vi "writeNumberOfImagesXML.vi"(8 "error in (no error)":errorcluster, 10 "NativeXML in":refnum<class "NativeXML.lvclass">, 11 "WinX32Settings in":refnum<class "WinX32Settings.lvclass">) -> (0 "error out":errorcluster, 2 "NativeXML out":refnum<class "NativeXML.lvclass">, 3 "WinX32Settings out":refnum<class "WinX32Settings.lvclass">)   [LabVIEW 2011, in "Tools.lvlib" / "Settings.lvlib" / "WinX32Settings.lvclass"]
uses:
  WinX32Settings.lvclass
  NativeXML/NativeXML.lvclass
  WinX32Settings.lvclass/WinX32Settings.ctl
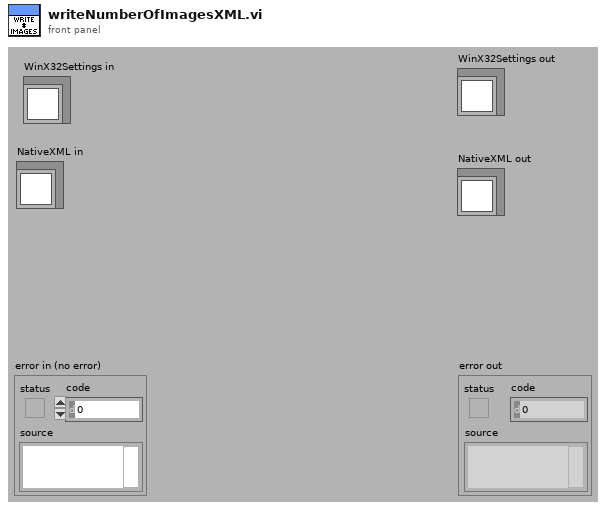
[diagram p1: front panel]
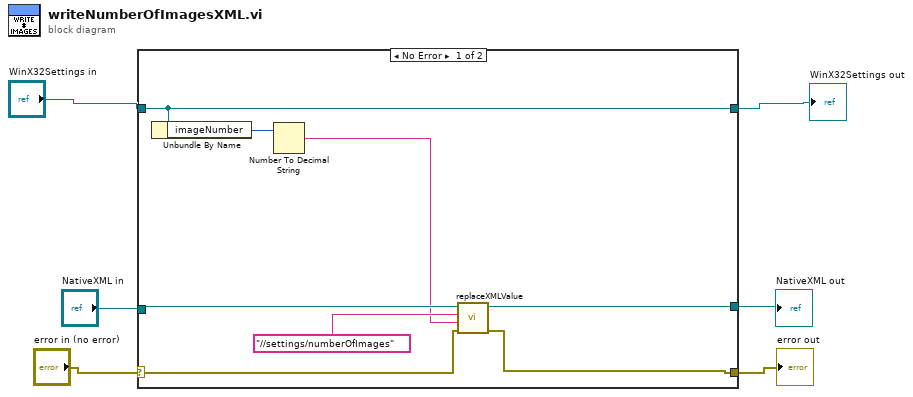
[diagram p0: block diagram]
diagram:
  n1 = case shown="No Error" "error in (no error)" {
    selector: "error in (no error)" -> [w10 w17]
    tunnel: [w9 w17] -> w6
    tunnel: [w14 w16] -> w1
    tunnel: "WinX32Settings in" -> [w14 w16]
    tunnel: "NativeXML in" -> [w13 w15]
    tunnel: [w12 w15] -> w5
    frame No Error {
      n2 = Unbundle By Name(w14) -> ("imageNumber"=w8:i32)
      n3 = Number To Decimal String(number=w8) -> (decimal integer string=w7:string)  [unwired: 1 in]
      n4 = call "replaceXMLValue.vi"("error in (no error)"=w10, "value"=w7, "replace in"="//settings/numberOfImages", "NativeXML in"=w13) -> ("error out"=w9:errorcluster, "NativeXML out"=w12:refnum<class "NativeXML.lvclass">)  [unwired: 6 in]
    }
    frame Error {
    }
  }
  "error out" <- w6
  "NativeXML out" <- w5
  "WinX32Settings out" <- w1
